vi "test_pixmap.vi"() -> ()   [LabVIEW 2010]
panel:
  out "Class Name":string
  out "Class ID":u32
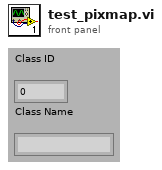
[diagram p1: front panel]
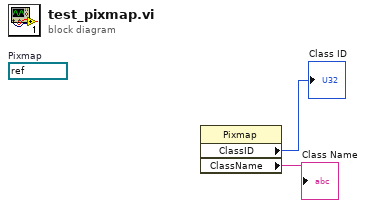
[diagram p0: block diagram]
diagram:
  (unwired) refnum<vi> refnum  # Pixmap
  n1 = property class="Pixmap"() -> ("ClassID"=→"Class ID":u32, "ClassName"=→"Class Name":string)  [unwired: 2 in, 2 out]
